vi "WF1974-rw_legacy.vi"(7 "Rotating Electric field":T1={"Start Frequency"=1000000.0, "Stop Frequency"=1000000.0, "Sweep Time"=10.0, "Amplitude"=4.0, "Phase (ch.1)"=90.0, "Phase (Ch.2)"=0.0} {"Sweep Time" format="%.4f"; "Phase (Ch.2)" min=-1800.0 max=1800.0 step=0.1 format="%.3f"; "Phase (ch.1)" min=-1800.0 max=1800.0 step=0.1 format="%.3f"; "Stop Frequency" format="%^.5e"; "Start Frequency" format="%^.5e"; "Amplitude" min=0.0 max=4.0 format="%.3f"}, 8 "error in (no error)":errorcluster caption="Error IN", 11 "VISAsession":refnum<visa-resource-name>="GPIB0::4::INSTR") -> (0 "error out":errorcluster caption="Error OUT", 3 "CopyVISAsession":refnum<visa-resource-name>="GPIB0::4::INSTR")   [LabVIEW 2018]
panel:
  out "x-y":dbl
  out "concatenated string":string
  # "manually set to 2-phase, sweep, 50 ohms"
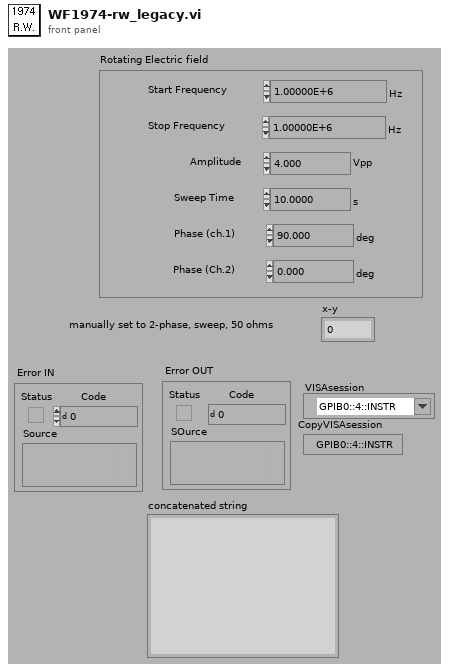
[diagram p1: front panel]
types:
  T1 = cluster{"Start Frequency":dbl, "Stop Frequency":dbl, "Sweep Time":dbl, "Amplitude":dbl, "Phase (ch.1)":dbl, "Phase (Ch.2)":dbl}
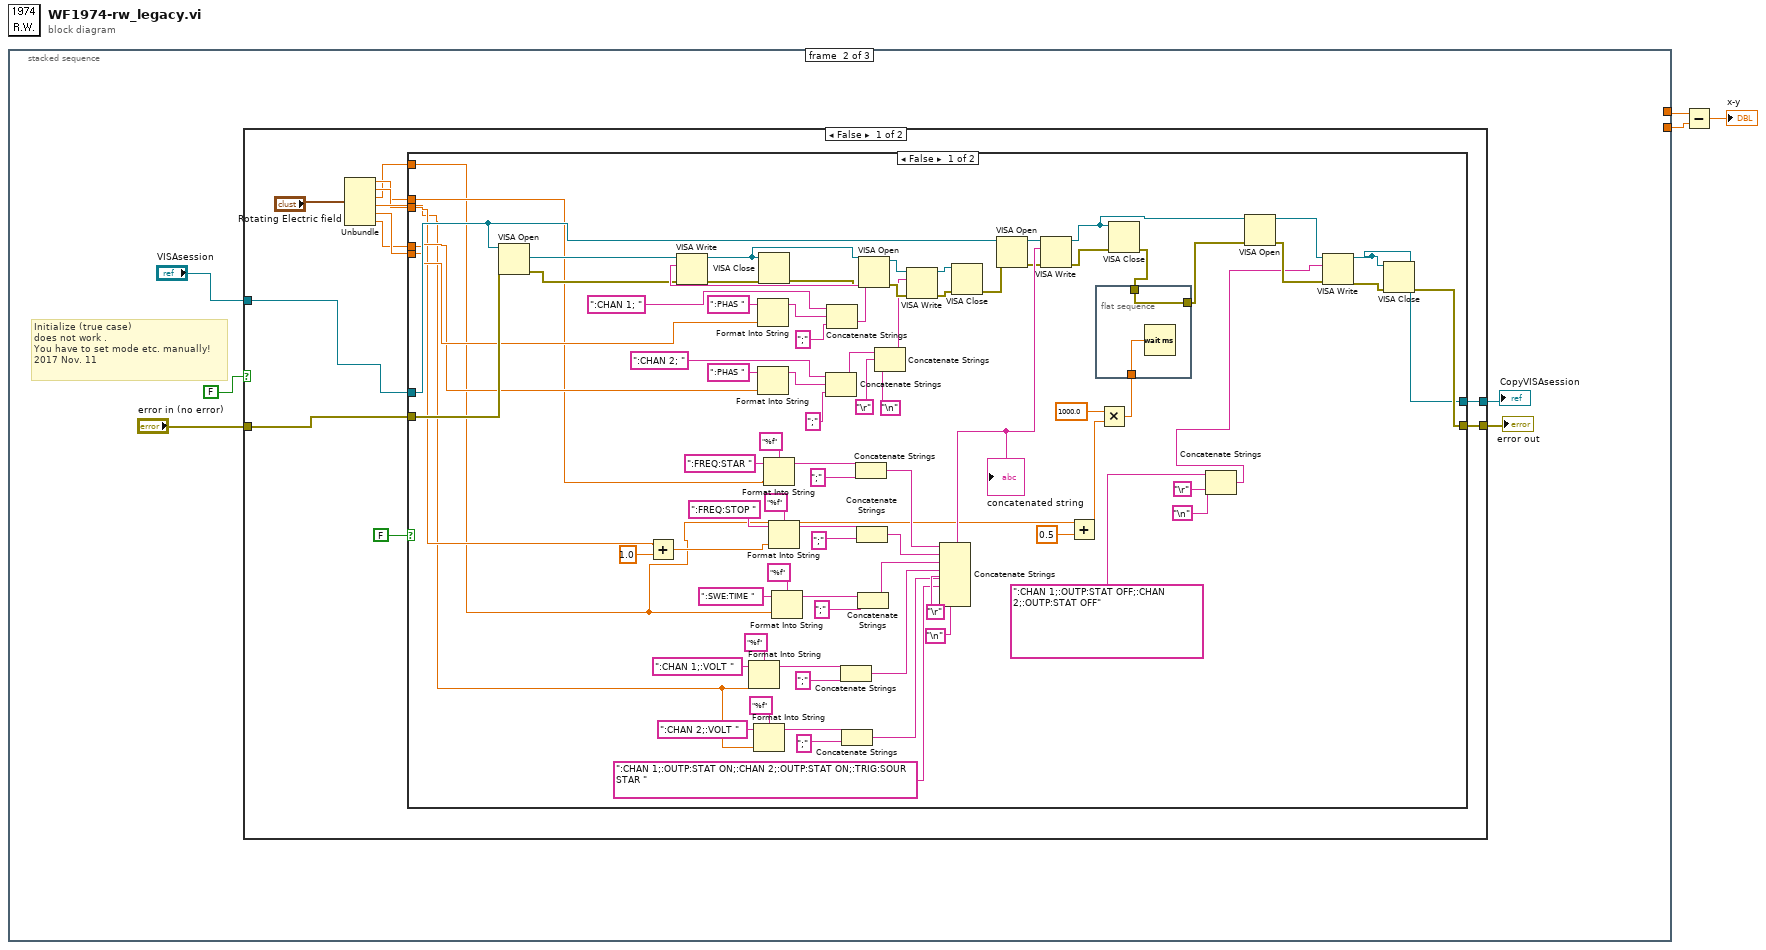
[diagram p0: block diagram]
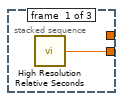
[diagram p2: hidden frame]
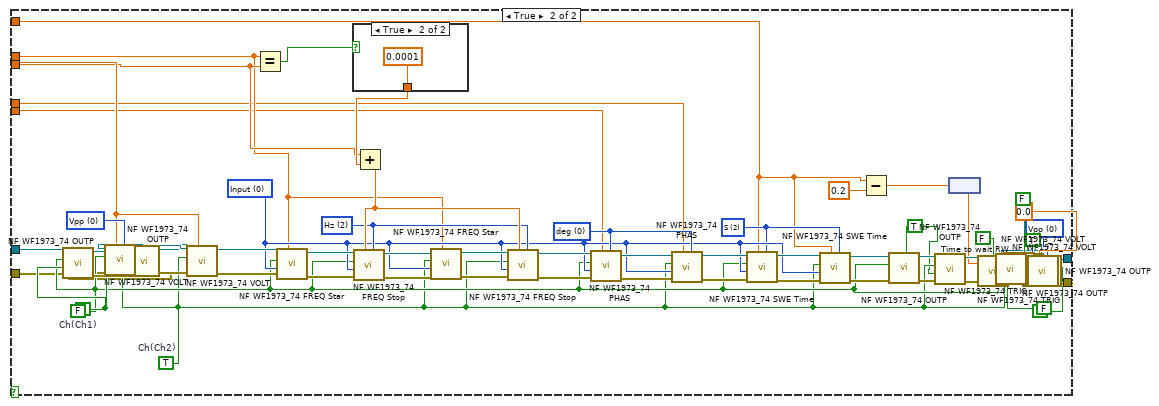
[diagram p3: hidden frame]
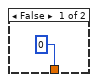
[diagram p4: hidden frame]
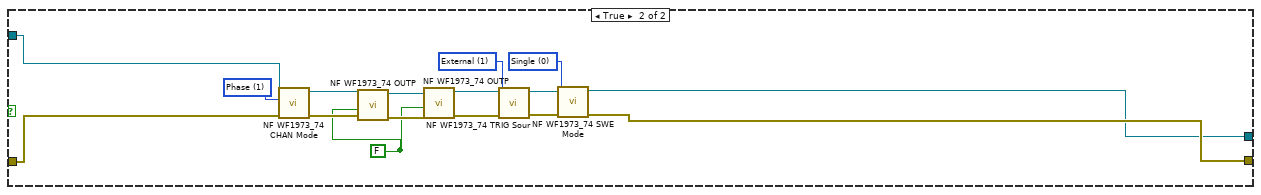
[diagram p5: hidden frame]
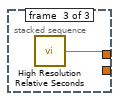
[diagram p6: hidden frame]
diagram:
  n1 = stacked-sequence {
    tunnel: [w4 _ _] -> w2
    tunnel: [_ _ w194] -> w3
    frame #0 {
      n2 = call <vilib>:"High Resolution Relative Seconds.vi"() -> ("relative seconds"=w4:dbl)
    }
    frame #1 {
      # "Initialize (true case)\ndoes not work .\nYou have to set mode etc. manually!\n2017 Nov. 11"
      n3 = case shown="False" FALSE ("Initialize ?") {
        tunnel: "error in (no error)" -> [w21 w181]
        tunnel: [w12 w180] -> w8
        tunnel: [w11 w179] -> w7
        tunnel: "VISAsession" -> [w20 w178]
        frame False {
          n4 = Unbundle("Rotating Electric field") -> ("Start Frequency"=w16:dbl, "Stop Frequency"=w17:dbl, "Sweep Time"=w15:dbl, "Amplitude"=w18:dbl, "Phase (ch.1)"=w14:dbl, "Phase (Ch.2)"=w13:dbl)
          n5 = case shown="False" FALSE {
            tunnel: w21 -> [w40 w130]
            tunnel: w20 -> [w39 w127]
            tunnel: w18 -> [w27 w126]
            tunnel: w17 -> [w32 w125]
            tunnel: w16 -> [w30 w124]
            tunnel: w15 -> [w29 w123]
            tunnel: w14 -> [w35 w122]
            tunnel: w13 -> [w34 w121]
            tunnel: [w38 w117] -> w12
            tunnel: [w36 w113] -> w11
            frame False {
              n6 = VISA Open(error in (no error)=w40, VISA resource name=w39) -> (VISA resource name=w41:refnum<visa-resource-name>, error out=w42:errorcluster)  [unwired: 3 in]
              n7 = Add(x=w32, y=1.0) -> (x+y=w33:dbl)
              n8 = Format Into String(format string="%f", initial string=":CHAN 1;:VOLT ", w27) -> (resulting string=w59:string)  [unwired: 1 in, 1 out]
              n9 = Format Into String(format string="%f", initial string=":CHAN 2;:VOLT ", w27) -> (resulting string=w61:string)  [unwired: 1 in, 1 out]
              n10 = Format Into String(initial string=":PHAS " ("Input String"), w35) -> (resulting string=w87:string)  [unwired: 2 in, 1 out]
              n11 = Format Into String(initial string=":PHAS " ("Input String"), w34) -> (resulting string=w89:string)  [unwired: 2 in, 1 out]
              n12 = Format Into String(format string="%f", initial string=":FREQ:STAR ", w30) -> (resulting string=w48:string)  [unwired: 1 in, 1 out]
              n13 = Format Into String(format string="%f", initial string=":FREQ:STOP ", w33) -> (resulting string=w50:string)  [unwired: 1 in, 1 out]
              n14 = Format Into String(format string="%f", initial string=":SWE:TIME ", w29) -> (resulting string=w52:string)  [unwired: 1 in, 1 out]
              n15 = Concatenate Strings(":CHAN 2; " ("Input String"), w89, ";" ("Substring")) -> (w77:string)
              n16 = Concatenate Strings(":CHAN 1; " ("Input String"), w87, ";" ("Substring")) -> (w96:string)
              n17 = VISA Write(VISA resource name=w41, write buffer=w96, error in (no error)=w42) -> (VISA resource name out=w94:refnum<visa-resource-name>, error out=w91:errorcluster)  [unwired: 1 out]
              n18 = VISA Close(VISA resource name=w94, error in (no error)=w91) -> (error out=w92:errorcluster)
              n19 = Concatenate Strings(w59, ";") -> (w63:string)
              n20 = Concatenate Strings(w61, ";") -> (w64:string)
              n21 = Concatenate Strings(w48, ";") -> (w73:string)
              n22 = Concatenate Strings(w50, ";") -> (w72:string)
              n23 = Concatenate Strings(w52, ";") -> (w54:string)
              n24 = VISA Open(error in (no error)=w92, VISA resource name=w94) -> (VISA resource name=w95:refnum<visa-resource-name>, error out=w93:errorcluster)  [unwired: 3 in]
              n25 = Concatenate Strings(w77, "\r", "\n") -> (w80:string)
              n26 = VISA Write(VISA resource name=w95, write buffer=w80, error in (no error)=w93) -> (VISA resource name out=w81:refnum<visa-resource-name>, error out=w82:errorcluster)  [unwired: 1 out]
              n27 = Concatenate Strings(w73, w72, w54, w63, w64, ":CHAN 1;:OUTP:STAT ON;:CHAN 2;:OUTP:STAT ON;:TRIG:SOUR STAR ", "\r", "\n") -> (w86:string)
              "concatenated string" <- w86
              n28 = VISA Close(VISA resource name=w81, error in (no error)=w82) -> (error out=w83:errorcluster)
              n29 = VISA Open(error in (no error)=w83, VISA resource name=w39) -> (VISA resource name=w84:refnum<visa-resource-name>, error out=w85:errorcluster)  [unwired: 3 in]
              n30 = VISA Write(VISA resource name=w84, write buffer=w86, error in (no error)=w85) -> (VISA resource name out=w101:refnum<visa-resource-name>, error out=w99:errorcluster)  [unwired: 1 out]
              n31 = Add(x=w29, y=0.5) -> (x+y=w24:dbl)
              n32 = flat-sequence {
                tunnel: w26 -> [w104]
                tunnel: [w104] -> w25
                tunnel: w22 -> [w103]
                frame #0 {
                  n33 = Wait (ms)(milliseconds to wait=w103) -> ()  [unwired: 1 out]
                }
              }
              n34 = Multiply(x=1000.0, y=w24) -> (x*y=w22:dbl)
              n35 = VISA Close(VISA resource name=w101, error in (no error)=w99) -> (error out=w26:errorcluster)
              n36 = Concatenate Strings(":CHAN 1;:OUTP:STAT OFF;:CHAN 2;:OUTP:STAT OFF", "\r", "\n") -> (w69:string)
              n37 = VISA Open(error in (no error)=w25, VISA resource name=w101) -> (VISA resource name=w102:refnum<visa-resource-name>, error out=w100:errorcluster)  [unwired: 3 in]
              n38 = VISA Write(VISA resource name=w102, write buffer=w69, error in (no error)=w100) -> (VISA resource name out=w36:refnum<visa-resource-name>, error out=w37:errorcluster)  [unwired: 1 out]
              n39 = VISA Close(VISA resource name=w36, error in (no error)=w37) -> (error out=w38:errorcluster)
            }
            frame True {
              w116 = 0.0 ("Amplitude(1)")
              w115 = u16 0 items=["Vpp", "Vpk", "Vrms", "dBv", "dBm", "USER", "mVpp", "mVpk", "mVrms"] ("Units(Vpp)")
              w131 = FALSE ("Output(OFF)")
              w134 = TRUE ("Output(OFF)")
              w147 = u16 2 items=["Mega(M)", "Kilo(k)", "S", "Milli(m)", "Micro(u)", "Nano(n)"] ("Units(S)")
              w153 = FALSE ("Output(OFF)")
              w156 = u16 0 items=["deg", "USER"] ("Units(deg)")
              w148 = u16 0 items=["Input", "Minimum", "Maximum"] ("Set Frequency(Input)")
              w165 = u16 2 items=["Mega(M)", "Kilo(k)", "Hz", "Micro(u)", "Nano(n)", "USER"] ("Units(Hz)")
              w173 = u16 0 items=["Vpp", "Vpk", "Vrms", "dBv", "dBm", "USER", "mVpp", "mVpk", "mVrms"] ("Units(Vpp)")
              w135 = TRUE  # Ch(Ch2)
              w136 = FALSE  # Ch(Ch1)
              n40 = call "NF WF1973_74 OUTP.vi"("error in (no error)"=w130, "Output(OFF)"=w153, "Ch(Ch1)"=w136, "VISAsession"=w127) -> ("error out"=w154:errorcluster, "CopyVISAsession"=w155:refnum<visa-resource-name>)  [unwired: 1 in, 5 out]
              n41 = call "NF WF1973_74 OUTP.vi"("error in (no error)"=w154, "Output(OFF)"=w153, "Ch(Ch1)"=w135, "VISAsession"=w155) -> ("error out"=w128:errorcluster, "CopyVISAsession"=w129:refnum<visa-resource-name>)  [unwired: 1 in, 5 out]
              n42 = call "NF WF1973_74 VOLT .vi"("Units(Vpp)"=w173, "Amplitude(1)"=w126, "error in (no error)"=w128, "Ch(Ch1)"=w136, "VISAsession"=w129) -> ("error out"=w174:errorcluster, "CopyVISAsession"=w175:refnum<visa-resource-name>)  [unwired: 2 in, 3 out]
              n43 = call "NF WF1973_74 VOLT .vi"("Amplitude(1)"=w126, "error in (no error)"=w174, "Ch(Ch1)"=w135, "VISAsession"=w175) -> ("error out"=w170:errorcluster, "CopyVISAsession"=w164:refnum<visa-resource-name>)  [unwired: 3 in, 3 out]
              n44 = Equal?(x=w124, y=w125) -> (x = y?=w172:bool)
              n45 = call "NF WF1973_74 FREQ Star.vi"("Frequency(1)"=w124, "error in (no error)"=w170, "Set Frequency(Input)"=w148, "Ch(Ch1)"=w136, "VISAsession"=w164) -> ("error out"=w169:errorcluster, "CopyVISAsession"=w163:refnum<visa-resource-name>)  [unwired: 2 in, 3 out]
              n46 = case shown="True" w172 {
                tunnel: [0 0.0001] -> w171
                frame False {
                }
                frame True {
                }
              }
              n47 = Add(x=w125, y=w171) -> (x+y=w166:dbl)
              n48 = call "NF WF1973_74 FREQ Stop.vi"("Units(Hz)"=w165, "Frequency(1)"=w166, "error in (no error)"=w169, "Set Frequency(Input)"=w148, "Ch(Ch1)"=w136, "VISAsession"=w163) -> ("error out"=w168:errorcluster, "CopyVISAsession"=w162:refnum<visa-resource-name>)  [unwired: 1 in, 3 out]
              n49 = call "NF WF1973_74 FREQ Star.vi"("Frequency(1)"=w124, "error in (no error)"=w168, "Set Frequency(Input)"=w148, "Ch(Ch1)"=w135, "VISAsession"=w162) -> ("error out"=w167:errorcluster, "CopyVISAsession"=w161:refnum<visa-resource-name>)  [unwired: 2 in, 3 out]
              n50 = call "NF WF1973_74 FREQ Stop.vi"("Units(Hz)"=w165, "Frequency(1)"=w166, "error in (no error)"=w167, "Set Frequency(Input)"=w148, "Ch(Ch1)"=w135, "VISAsession"=w161) -> ("error out"=w159:errorcluster, "CopyVISAsession"=w160:refnum<visa-resource-name>)  [unwired: 1 in, 3 out]
              n51 = call "NF WF1973_74 PHAS.vi"("Units(deg)"=w156, "Phase(0)"=w122, "error in (no error)"=w159, "Set Phase(Input)"=w148, "Ch(Ch1)"=w136, "VISAsession"=w160) -> ("error out"=w158:errorcluster, "CopyVISAsession"=w157:refnum<visa-resource-name>)  [unwired: 1 in, 3 out]
              n52 = call "NF WF1973_74 PHAS.vi"("Units(deg)"=w156, "Phase(0)"=w121, "error in (no error)"=w158, "Set Phase(Input)"=w148, "Ch(Ch1)"=w135, "VISAsession"=w157) -> ("error out"=w152:errorcluster, "CopyVISAsession"=w150:refnum<visa-resource-name>)  [unwired: 1 in, 3 out]
              n53 = call "NF WF1973_74 SWE Time.vi"("Units(S)"=w147, "Time(1)"=w123, "error in (no error)"=w152, "Set Time(Input)"=w148, "Ch(Ch1)"=w136, "VISAsession"=w150) -> ("error out"=w151:errorcluster, "CopyVISAsession"=w149:refnum<visa-resource-name>)  [unwired: 1 in, 3 out]
              n54 = call "NF WF1973_74 SWE Time.vi"("Units(S)"=w147, "Time(1)"=w123, "error in (no error)"=w151, "Set Time(Input)"=w148, "Ch(Ch1)"=w135, "VISAsession"=w149) -> ("error out"=w145:errorcluster, "CopyVISAsession"=w140:refnum<visa-resource-name>)  [unwired: 1 in, 3 out]
              n55 = Subtract(x=w123, y=0.2) -> (x-y=w133:dbl)
              n56 = call "NF WF1973_74 OUTP.vi"("error in (no error)"=w145, "Output(OFF)"=w134, "Ch(Ch1)"=w136, "VISAsession"=w140) -> ("error out"=w144:errorcluster, "CopyVISAsession"=w139:refnum<visa-resource-name>)  [unwired: 1 in, 5 out]
              n57 = call "NF WF1973_74 OUTP.vi"("error in (no error)"=w144, "Output(OFF)"=w134, "Ch(Ch1)"=w135, "VISAsession"=w139) -> ("error out"=w143:errorcluster, "CopyVISAsession"=w138:refnum<visa-resource-name>)  [unwired: 1 in, 5 out]
              n58 = node(w133) -> (w132:dbl[unit])
              n59 = call "NF WF1973_74 TRIG.vi"("error in (no error)"=w143, "Ch(Ch1)"=FALSE, "VISAsession"=w138) -> ("error out"=w110:errorcluster, "CopyVISAsession"=w107:refnum<visa-resource-name>)  [unwired: 7 out]
              n60 = call "NF WF1973_74 TRIG.vi"("error in (no error)"=w110, "Ch(Ch1)"=TRUE, "VISAsession"=w107) -> ("error out"=w109:errorcluster, "CopyVISAsession"=w108:refnum<visa-resource-name>)  [unwired: 7 out]
              n61 = call "Time to wait RW.vi"("error in (no error)"=w109, "Time to wait"=w132) -> ("error out"=w142:errorcluster)
              n62 = call "NF WF1973_74 OUTP.vi"("error in (no error)"=w142, "Output(OFF)"=w131, "Ch(Ch1)"=w136, "VISAsession"=w108) -> ("error out"=w141:errorcluster, "CopyVISAsession"=w137:refnum<visa-resource-name>)  [unwired: 1 in, 5 out]
              n63 = call "NF WF1973_74 OUTP.vi"("error in (no error)"=w141, "Output(OFF)"=w131, "Ch(Ch1)"=w135, "VISAsession"=w137) -> ("error out"=w120:errorcluster, "CopyVISAsession"=w119:refnum<visa-resource-name>)  [unwired: 1 in, 5 out]
              n64 = call "NF WF1973_74 VOLT .vi"("Units(Vpp)"=w115, "Amplitude(1)"=w116, "error in (no error)"=w120, "Ch(Ch1)"=FALSE, "VISAsession"=w119) -> ("error out"=w112:errorcluster, "CopyVISAsession"=w114:refnum<visa-resource-name>)  [unwired: 2 in, 3 out]
              n65 = call "NF WF1973_74 VOLT .vi"("Units(Vpp)"=w115, "Amplitude(1)"=w116, "error in (no error)"=w112, "Ch(Ch1)"=TRUE, "VISAsession"=w114) -> ("error out"=w117:errorcluster, "CopyVISAsession"=w113:refnum<visa-resource-name>)  [unwired: 2 in, 3 out]
            }
          }
        }
        frame True {
          w193 = u16 0 items=["Single", "Continue", "Gated"] ("Mode (Single)")
          w182 = 1 items=["Independent", "Phase", "Tone", "Ratio", "Differential"] ("Channel Mode(Independent)")
          w183 = FALSE ("Output(OFF)")
          w192 = u32 1 items=["Timer", "External", "CH1"] ("Source(Timer)")
          n66 = call "NF WF1973_74 CHAN Mode.vi"("error in (no error)"=w181, "Channel Mode(Independent)"=w182, "VISAsession"=w178) -> ("error out"=w186:errorcluster, "CopyVISAsession"=w189:refnum<visa-resource-name>)  [unwired: 1 in, 6 out]
          n67 = call "NF WF1973_74 OUTP.vi"("error in (no error)"=w186, "Output(OFF)"=w183, "VISAsession"=w189) -> ("error out"=w185:errorcluster, "CopyVISAsession"=w188:refnum<visa-resource-name>)  [unwired: 2 in, 5 out]
          n68 = call "NF WF1973_74 OUTP.vi"("error in (no error)"=w185, "Output(OFF)"=w183, "VISAsession"=w188) -> ("error out"=w184:errorcluster, "CopyVISAsession"=w187:refnum<visa-resource-name>)  [unwired: 2 in, 5 out]
          n69 = call "NF WF1973_74 TRIG Sour.vi"("error in (no error)"=w184, "Source(Timer)"=w192, "VISAsession"=w187) -> ("error out"=w190:errorcluster, "CopyVISAsession"=w191:refnum<visa-resource-name>)  [unwired: 3 in, 4 out]
          n70 = call "NF WF1973_74 SWE Mode.vi"("error in (no error)"=w190, "Mode (Single)"=w193, "VISAsession"=w191) -> ("error out"=w180:errorcluster, "CopyVISAsession"=w179:refnum<visa-resource-name>)  [unwired: 2 in, 5 out]
        }
      }
      "error out" <- w8
      "CopyVISAsession" <- w7
    }
    frame #2 {
      n71 = call <vilib>:"High Resolution Relative Seconds.vi"() -> ("relative seconds"=w194:dbl)
    }
  }
  n72 = Subtract(x=w3, y=w2) -> (x-y=→"x-y":dbl)
